vi "Send Log Data.vi"(8 "error in":errorcluster, 10 "Data":T1[](array[typedef]) {"type" format="%04x"; "activity" format="%04x"; "error" format="%04x"; "cwd1" format="%04x"; "cwd2" format="%04x"; "swd1" format="%04x"; "swd2" format="%04x"; "data" format="%04x"}, 11 "Log Producer in":refnum<class "Log Producer.lvclass">) -> (0 "error out":errorcluster, 3 "Log Producer out":refnum<class "Log Producer.lvclass">)   [LabVIEW 2023, in "Ballard MIL-STD-1553 Engine Support.lvlib" / "Implementation.lvlib" / "Word Logging.lvlib" / "Log Producer.lvclass"]
uses:
  Log Producer.lvclass
  Word.ctl
  Log Producer.lvclass/Log Producer.ctl
  Log Message/Log Message.lvclass
  C:/Program Files/National Instruments/LabVIEW 2023/vi.lib/NI/VeriStand Custom Device Messaging/Message/Abstract Message/Abstract Message.lvclass
  Implementation.lvlib
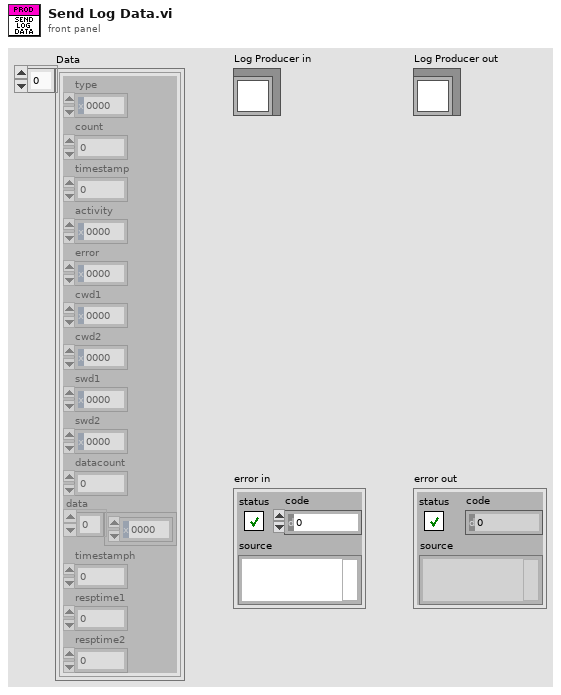
[diagram p1: front panel]
types:
  T1 = typedef "Ballard MIL-STD-1553 Engine Support.lvlib/Implementation.lvlib/Word.ctl" = cluster{"type":u16, "count":u16, "timestamp":u32, "activity":u16, "error":u16, "cwd1":u16, "cwd2":u16, "swd1":u16, "swd2":u16, "datacount":u16, "data":u16[], "timestamph":u32, "resptime1":u16, "resptime2":u16}
  T2 = typedef "Ballard MIL-STD-1553 Engine Support.lvlib/Implementation.lvlib/Word Logging.lvlib/Logger Data Reference.ctl" = refnum<data-value>
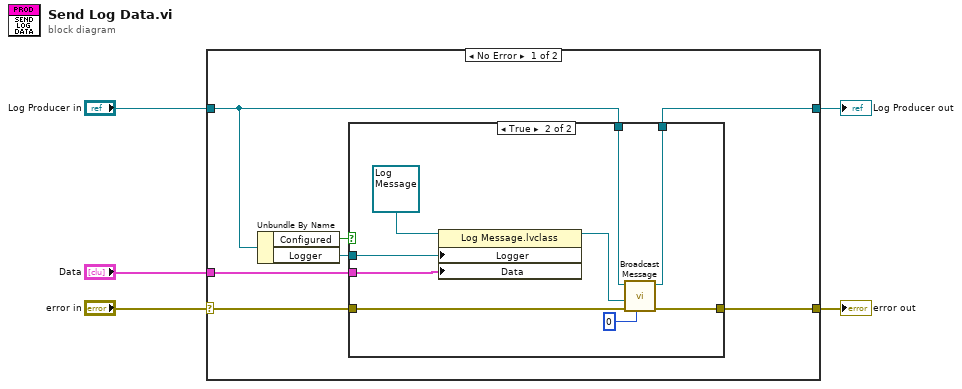
[diagram p0: block diagram]
diagram:
  n1 = case shown="No Error" "error in" {
    selector: "error in" -> [w11 w25]
    tunnel: [w10 w25] -> w4
    tunnel: [w8 w24] -> w2
    tunnel: "Log Producer in" -> [w9 w24]
    tunnel: "Data" -> [w7 _]
    frame No Error {
      n2 = Unbundle By Name(w9) -> ("Configured"=w6:bool, "Logger"=w12:T2)
      n3 = case shown="True" w6 {
        tunnel: w12 -> [_ w23]
        tunnel: w11 -> [w13 w22]
        tunnel: [w13 w21] -> w10
        tunnel: w9 -> [w14 w20]
        tunnel: [w14 w19] -> w8
        tunnel: w7 -> [_ w16]
        frame False {
        }
        frame True {
          n4 = property class="Log Message.lvclass"(reference=refnum<class "Log Message.lvclass"> refnum ("Communication Bus Template Interfaces:Implementation.lvlib:Logging.lvlib:Log Word Message.lvclass"), "Logger"=w23, "Data"=w16) -> (reference out=w18:refnum<class "Log Message.lvclass">)  [unwired: 1 in, 1 out]
          n5 = call-dynamic "Broadcast Message.vi"("timeout in ms (-1)"=0, "error in (no error)"=w22, "Message in"=w18, "Abstract Producer in"=w20) -> ("error out"=w21:errorcluster, "Abstract Producer out"=w19:refnum<class "Log Producer.lvclass">)  [unwired: 4 in, 2 out]
        }
      }
    }
    frame Error {
    }
  }
  "error out" <- w4
  "Log Producer out" <- w2
